vi "cmd_quit.vi"(8 "error in (no error)":errorcluster, 11 "JSON":string) -> (0 "error out":errorcluster)   [LabVIEW 2021]
doc: "Exit the system"
uses:
  core/host_global_vars.vi
  <vilib>/Utility/error.llb/Error Cluster From Error Code.vi
  <vilib>/rvi/errors/niLvFpgaAdjustHostInterfaceError.vi
  <vilib>/rvi/interface/nirviReadWriteControl/nirviReadWriteControl.xnode
  FPGA Bitfiles/openlabspm_FPGATarget_fpgamain_eo-gUZR5D1g.lvbitx
  fpga/fpga_main.vi
  NiFpgaLv.dll
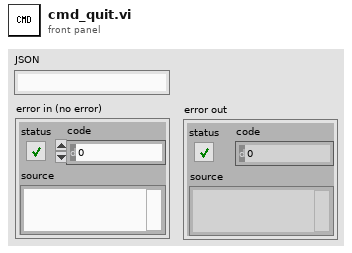
[diagram p1: front panel]
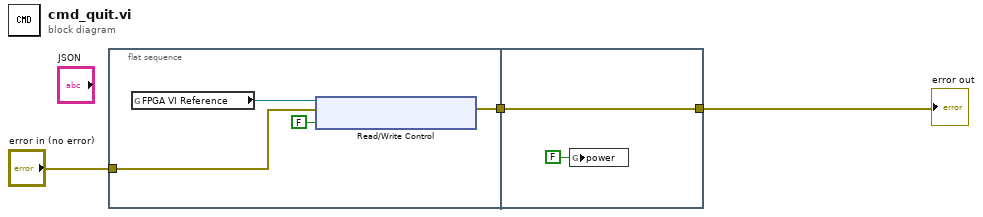
[diagram p0: block diagram]
diagram:
  n1 = flat-sequence {
    tunnel: "error in (no error)" -> [w6]
    tunnel: [w4] -> w2
    tunnel: [w9] -> w1
    tunnel: w2 -> [w9]
    frame #0 {
      n2 = global read "host_global_vars.vi" "FPGA VI Reference"() -> (w7:refnum<k20>)
      n3 = xnode "Read/Write Control"("FPGA VI Reference In"=w7, "error in"=w6, "DMA"=FALSE) -> ("error out"=w4:errorcluster)  [unwired: 1 out]
    }
    frame #1 {
      n4 = global write "host_global_vars.vi" "power"(FALSE ("power")) -> ()
    }
  }
  "error out" <- w1
